vi "MI Attributes.vi"(10 "MI Terms":i32[](array[numeric])) -> (1 "Read MI":i32[](array[numeric]), 2 "Init MI":i32[](array[numeric]))   [LabVIEW 2025, in "_Rescript.lvlib" / "Msg.lvlib"]
uses:
  Msg.lvlib
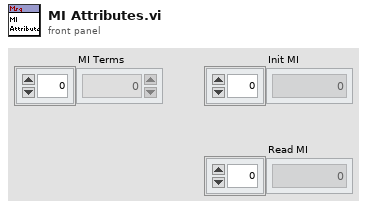
[diagram p1: front panel]
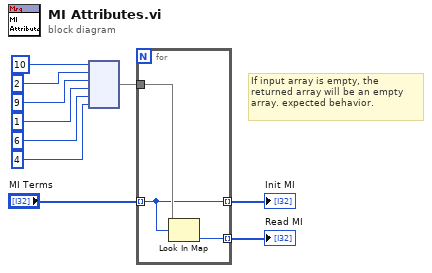
[diagram p0: block diagram]
diagram:
  # "If input array is empty, the returned array will be an empty array. expected behavior."
  n1 = node(10 ("Numeric"), 2 ("Numeric"), 9 ("Numeric"), 1 ("Numeric"), 6 ("key"), 4 ("value")) -> (w4:map{i32, i32})
  n2 = for {
    tunnel: [w12] -> w10 mode=indexing
    tunnel: "MI Terms" -> [w12] mode=indexing
    tunnel: w4 -> [w13]
    tunnel: [w11] -> w3 mode=indexing
    n3 = Look In Map(map=w13, key=w12) -> (value=w11:i32)  [unwired: 1 in, 1 out]
  }
  "Init MI" <- w10
  "Read MI" <- w3
